vi "Config Trig Window.vi"(0 "VISA resource name":refnum<visa-resource-name>, 5 "Condition(F: In)":bool, 7 "Center Level (0)":dbl min=-100.0 max=100.0 step=0.10000000149011612 format="%.1f", 9 "Window Width (25.0)":dbl=25.0 min=0.0 max=200.0 step=0.10000000149011612 format="%.1f", 11 "error in (no error)":errorcluster) -> (4 "VISA resource name out":refnum<visa-resource-name>, 15 "error out":errorcluster)   [LabVIEW 2013, in "Yokogawa.lvlib" / "Yokogawa PZ4000.lvlib"]
doc: "This VI sends the Trigger Control command to the PZ4000.\nConfiguration Functions are Condition, Center Level, and Window Width of Window Trigger."
uses:
  Yokogawa PZ4000.lvlib
panel:
  # "Out\nIn"
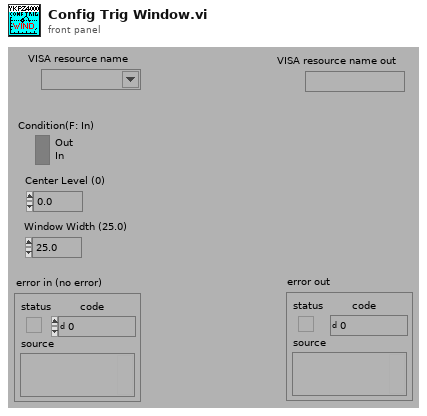
[diagram p1: front panel]
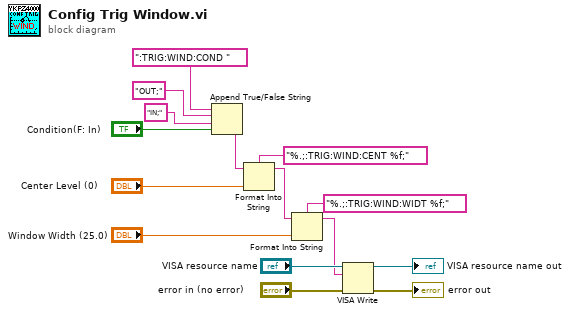
[diagram p0: block diagram]
diagram:
  n1 = Append True/False String(1:"Condition(F: In)", 2:"IN;", 3:"OUT;", 4:":TRIG:WIND:COND ") -> (0:w3:string)
  n2 = Format Into String(format string="%.;:TRIG:WIND:CENT %f;", initial string=w3, "Center Level (0)") -> (resulting string=w2:string)  [unwired: 1 in, 1 out]
  n3 = Format Into String(format string="%.;:TRIG:WIND:WIDT %f;", initial string=w2, "Window Width (25.0)") -> (resulting string=w1:string)  [unwired: 1 in, 1 out]
  n4 = VISA Write(VISA resource name="VISA resource name", write buffer=w1, error in (no error)="error in (no error)") -> (VISA resource name out=→"VISA resource name out":refnum<visa-resource-name>, error out=→"error out":errorcluster)  [unwired: 1 out]
